vi "Embed Image relative.vi"(8 "error in (no error)":errorcluster, 9 "imagename":string, 10 "Pict Refnum":refnum<vi>, 11 "Application path":path) -> (0 "error out":errorcluster)   [LabVIEW 2023, in "EmbedImage.lvlib" / "EmbedImage.lvclass"]
doc: "This routine will look for any legal image format of a specified name in the application directory, then insert it in to the provided reference."
uses:
  Library/EmbedImage.lvclass
  Library/EmbedImage.lvclass/EmbedImage.ctl
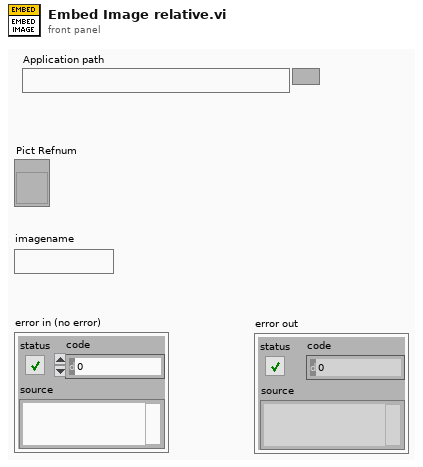
[diagram p1: front panel]
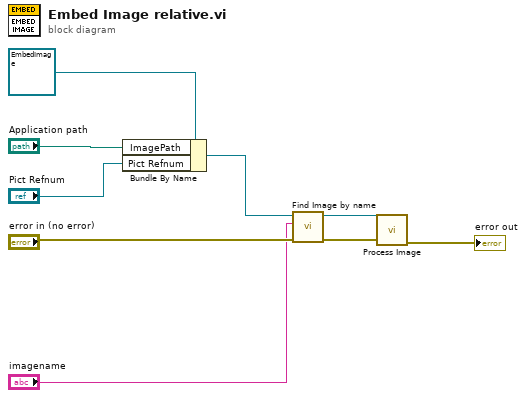
[diagram p0: block diagram]
diagram:
  n1 = Bundle By Name(cluster=refnum<class "EmbedImage.lvclass"> refnum ("EmbedImage.lvlib:EmbedImage.lvclass"), "ImagePath"="Application path", "Pict Refnum"="Pict Refnum") -> (w6:refnum<class "EmbedImage.lvclass">)
  n2 = call "Find Image by name.vi"("error in (no error)"="error in (no error)", "Imagename"="imagename", "EmbedImage in"=w6) -> ("error out"=w4:errorcluster, "EmbedImage out"=w5:refnum<class "EmbedImage.lvclass">)  [unwired: 7 in]
  n3 = call "Process Image.vi"("error in (no error)"=w4, "EmbedImage in"=w5) -> ("error out"=→"error out":errorcluster)  [unwired: 8 in, 1 out]
